vi "handleMessage.vi"(8 "error in (no error)":errorcluster, 11 "InputMessage":string) -> (0 "error out":errorcluster, 3 "OutputMessage":string)   [LabVIEW 2019]
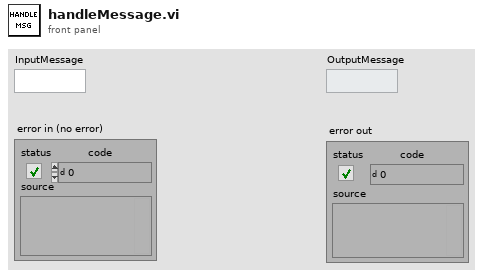
[diagram p1: front panel]
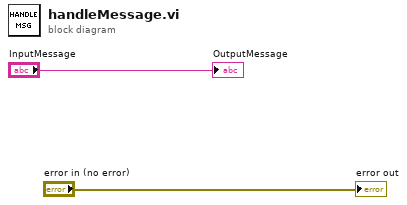
[diagram p0: block diagram]
diagram:
  "OutputMessage" <- "InputMessage"
  "error out" <- "error in (no error)"
